vi "Create Evaluations.vi"(8 "error in (no error)":errorcluster, 11 "IEvaluation in":refnum<class "Skyworks_LNA_Modeswitch.lvclass">) -> (0 "error out":errorcluster, 2 "Evaluations Out":T1[](array[typedef]) {"Low Limit" format="%#_13g"; "SI Scaling" items=["femto"=-15, "pico"=-12, "nano"=-9, "micro"=-6, "milli"=-3, "percent"=-2, ""=0, "kilo"=3, "mega"=6, "giga"=9, "tera"=12]}, 3 "IEvaluation out":refnum<class "Skyworks_LNA_Modeswitch.lvclass">)   [LabVIEW 2016, in "SeqAuto Evaluations.lvlib" / "Skyworks_LNA_Modeswitch.lvclass"]
uses:
  Skyworks_LNA_Modeswitch.lvclass
  C:/Sequence Automation/Plugins/SeqAuto IEvaluation.lvlibp/SeqAuto IEvaluation.lvclass
  Plugins/TestStand API Tools (TSAT).lvlibp/Evaluation Actions/Includes/Controls/TSAT Evaluation.ctl
  Plugins/TestStand API Tools (TSAT).lvlibp/Evaluation Actions/Includes/Controls/TSAT Eval SI Unit Scaling.ctl
  Plugins/TestStand API Tools (TSAT).lvlibp/Evaluation Actions/Includes/Controls/TSAT Evaluation Type.ctl
  Skyworks_LNA_Modeswitch.lvclass/Skyworks_LNA_Modeswitch.ctl
  Plugins/SeqAuto IEvaluation.lvlibp/Read Measurement Name.vi
  Plugins/TestStand API Tools (TSAT).lvlibp/Evaluation Actions/TSAT Evaluation Actions.lvlib
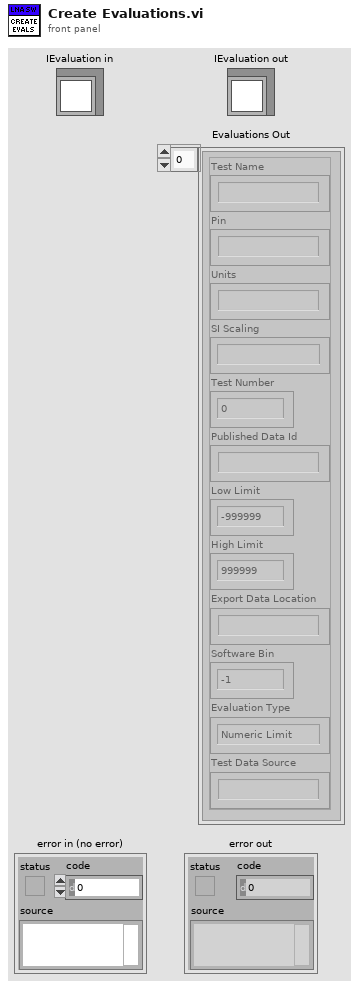
[diagram p1: front panel]
types:
  T1 = typedef "TestStand API Tools (TSAT).lvlibp/TSAT Evaluation Actions.lvlib/TSAT Evaluation.ctl" = cluster{"Test Name":string, "Pin":string, "Units":string, "SI Scaling":T2, "Test Number":i32, "Published Data Id":string, "Low Limit":dbl, "High Limit":dbl, "Export Data Location":string, "Software Bin":i64, "Evaluation Type":T3, "Test Data Source":string}
  T2 = typedef "TestStand API Tools (TSAT).lvlibp/TSAT Evaluation Actions.lvlib/TSAT Eval SI Unit Scaling.ctl" = i16
  T3 = typedef "TestStand API Tools (TSAT).lvlibp/TSAT Evaluation Actions.lvlib/TSAT Evaluation Type.ctl" = enum16{"Numeric Limit", "Pass/Fail", "None"}
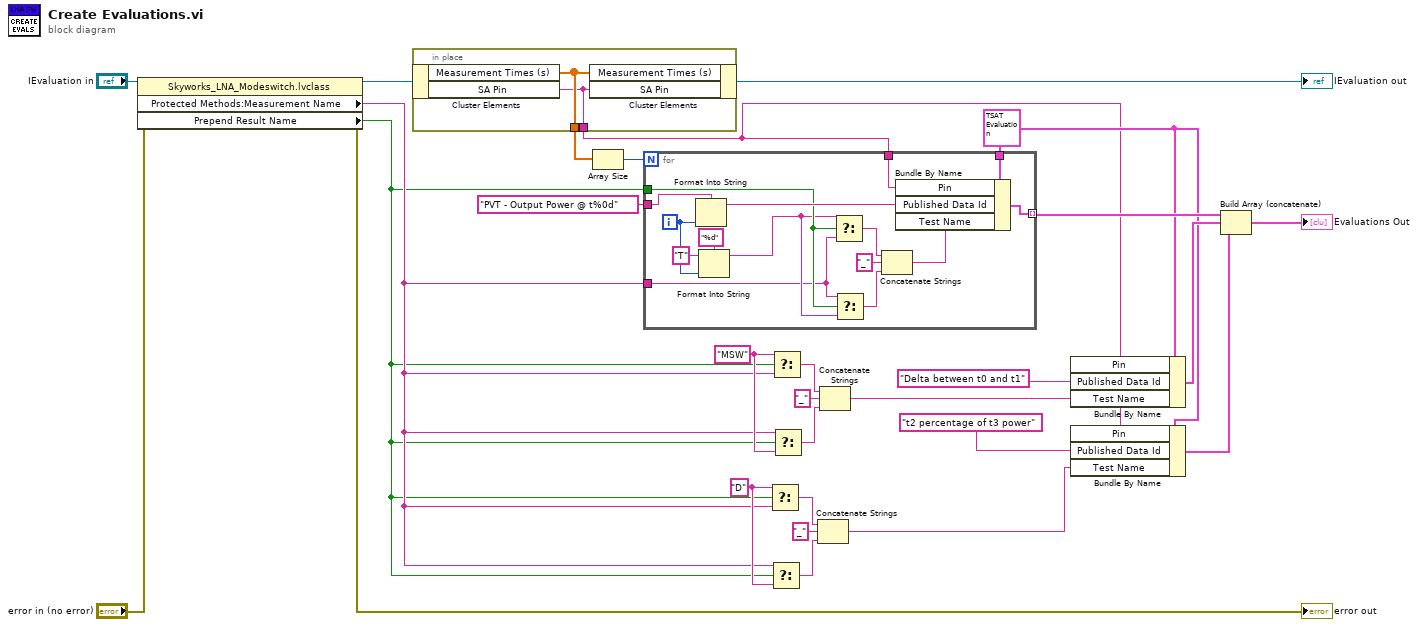
[diagram p0: block diagram]
diagram:
  w5 = "D" ("string")
  w18 = "MSW" ("string")
  w9 = T1 {"Test Name"="", "Pin"="", "Units"="", "SI Scaling"=0, "Test Number"=0, "Published Data Id"="", "Low Limit"=-999999.0, "High Limit"=999999.0, "Export Data Location"="", "Software Bin"=-1, "Evaluation Type"=enum."Numeric Limit", "Test Data Source"=""} ("Evaluation")
  n1 = property class="Skyworks_LNA_Modeswitch.lvclass"(reference="IEvaluation in", error in="error in (no error)") -> (reference out=w23:refnum<class "Skyworks_LNA_Modeswitch.lvclass">, error out=→"error out":errorcluster, "Protected Methods:Measurement Name"=w2:string, "Prepend Result Name"=w1:bool)
  n2 = in-place {
    in-place-border: [w30] -> w26
    in-place-border: [w29] -> w3
    n3 = in-place-cluster #1(w23) -> ("Measurement Times (s)"=w30:dbl[], "SA Pin"=w29:string)
    n4 = in-place-cluster #1("Measurement Times (s)"=w30, "SA Pin"=w29) -> (→"IEvaluation out":refnum<class "Skyworks_LNA_Modeswitch.lvclass">)
  }
  n5 = Array Size(array=w26) -> (size(s)=w24:i32)
  n6 = for {
    N: w24 -> [_]
    tunnel: "PVT - Output Power @ t%0d" -> [w33]
    tunnel: w9 -> [w45]
    tunnel: w2 -> [w31]
    tunnel: w1 -> [w39]
    tunnel: [w35] -> w16 mode=indexing
    tunnel: w3 -> [w34]
    i -> [w43]
    n7 = Format Into String(format string=w33, w43) -> (resulting string=w44:string)  [unwired: 2 in, 1 out]
    n8 = Format Into String(format string="%d", initial string="T", w43) -> (resulting string=w32:string)  [unwired: 1 in, 1 out]
    n9 = Select(t=w32, s=w39, f=w31) -> (s? t:f=w38:string)
    n10 = Select(t=w31, s=w39, f=w32) -> (s? t:f=w37:string)
    n11 = Concatenate Strings(w38, "_" ("string"), w37) -> (w36:string)
    n12 = Bundle By Name(cluster=w45, "Pin"=w34, "Published Data Id"=w44, "Test Name"=w36) -> (w35:T1)
  }
  n13 = Select(t=w5, s=w1, f=w2) -> (s? t:f=w7:string)
  n14 = Select(t=w2, s=w1, f=w5) -> (s? t:f=w6:string)
  n15 = Select(t=w18, s=w1, f=w2) -> (s? t:f=w20:string)
  n16 = Select(t=w2, s=w1, f=w18) -> (s? t:f=w19:string)
  n17 = Concatenate Strings(w7, "_" ("string"), w6) -> (w4:string)
  n18 = Concatenate Strings(w20, "_" ("string"), w19) -> (w17:string)
  n19 = Bundle By Name(cluster=w9, "Pin"=w3, "Published Data Id"="Delta between t0 and t1", "Test Name"=w17) -> (w15:T1)
  n20 = Bundle By Name(cluster=w9, "Pin"=w3, "Published Data Id"="t2 percentage of t3 power", "Test Name"=w4) -> (w10:T1)
  n21 = Build Array (concatenate)(w16, w15, w10) -> (→"Evaluations Out":T1[])
